vi "Tavle Save for PD.vi"(8 "error in (no error)":errorcluster, 11 "SN":string) -> (0 "error out":errorcluster, 3 "條碼的Index":i32)   [LabVIEW 2019]
uses:
  Ctrl/Table Save.ctl
  LLB/Message/Ctrl/LogType.ctl
  <vilib>/Utility/sysdir.llb/System Directory Type.ctl
  <vilib>/Utility/file.llb/Write Delimited Spreadsheet (string).vi
  LLB/Message/MsgShowAndLog.lvlib
panel:
  out "Read SN Table":string[][](array[string])
  in  "Base Path":path=path "D:/Vicomm"
  out "element":string
  in  "Cluster":cluster{"Table Control":string[][]}={"Table Control"=[["PCBA BARCODE", ""], ["硬體(Tool初始化)", ""], ["company(Tool初始化)", ""], ["耗電流 uA(電流表)", "T"], ["電池負載電壓", "T"], ["晶片ID(Tool FORMAT)", "F"], ["雷雕ID(TOOl scan、藍芽接收器)", "S"], ["Format(Tool FORMAT)", "F"], ["Programe(Tool Programe)", "P"]]}
  # "-1 : 未找到條碼"
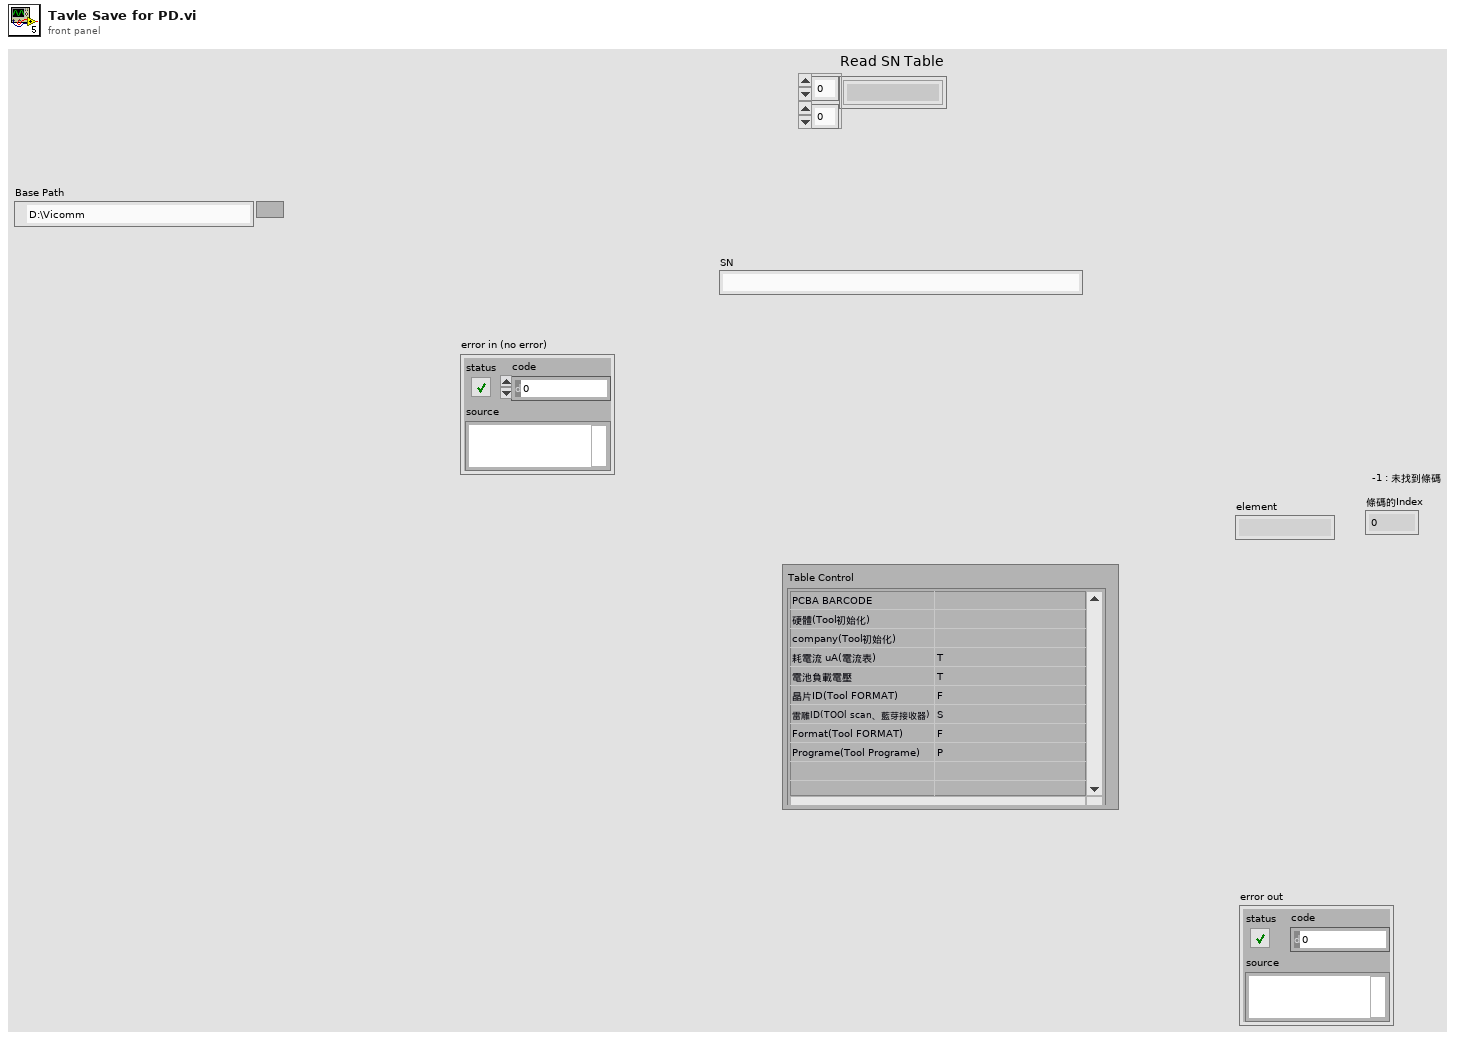
[diagram p1: front panel]
types:
  T1 = typedef "Table Save.ctl" = enum16{"initial", "Add", "Write", "Replace", "Delete", "REad", "RedTable", "Load"}
  T2 = enum16{"open", "replace", "create", "open or create", "replace or create", "replace or create with confirmation"}
  T3 = typedef "MsgShowAndLog.lvlib/LogType.ctl" = enum16{"Auto", "Manual", "Handshake", "Error"}
  T4 = typedef "System Directory Type.ctl" = i32
  T5 = typedef "LVDateTimeRec.ctl" = cluster{"fractional second":dbl, "second":i32, "minute":i32, "hour":i32, "day of month":i32, "month":i32, "year":i32, "day of week":i32, "day of year":i32, "DST":i32}
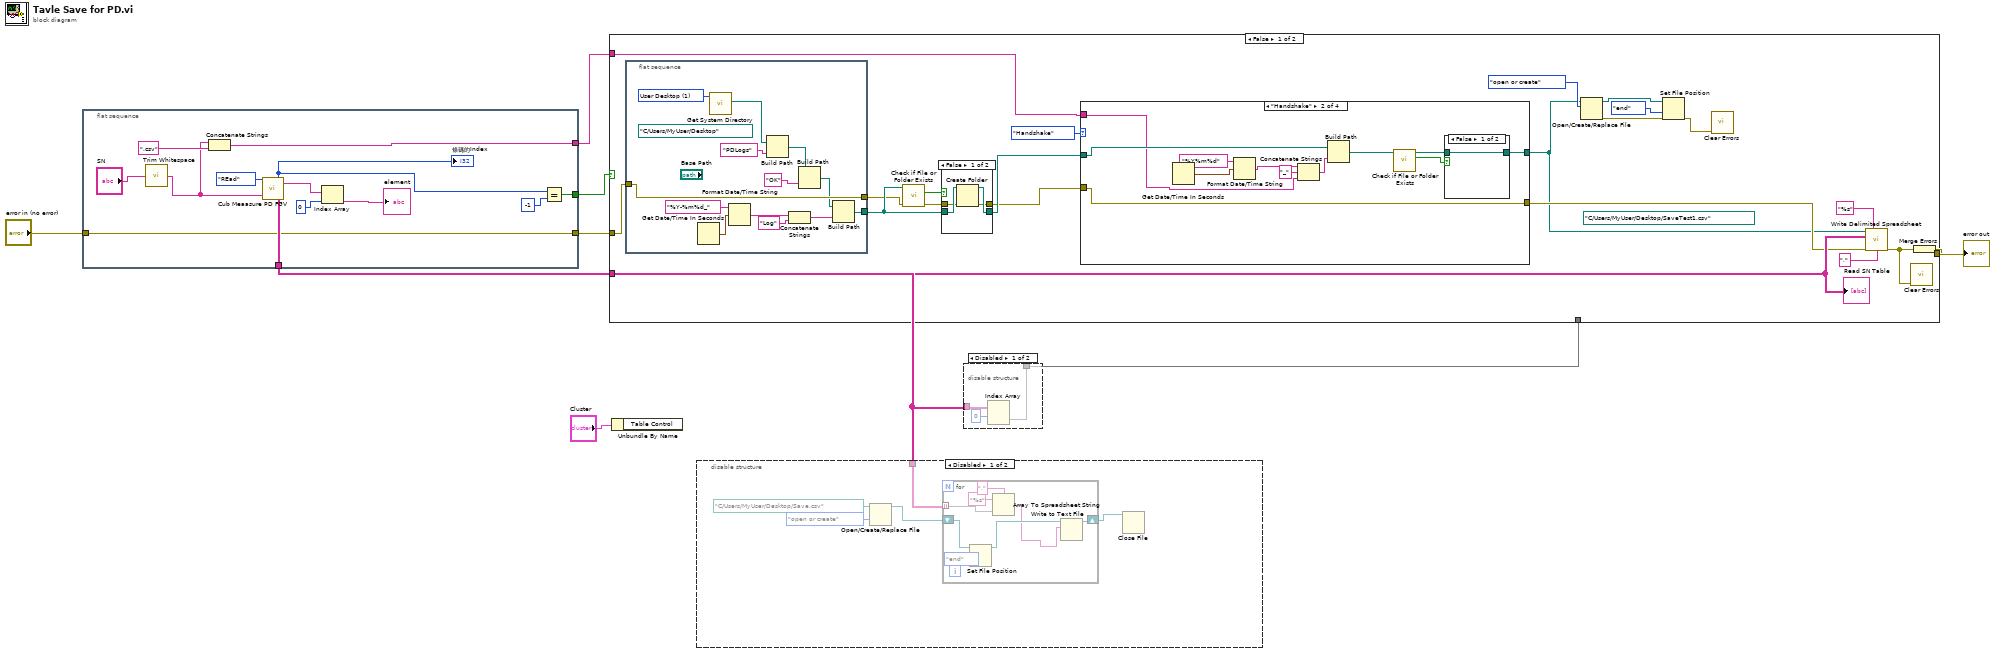
[diagram p0: block diagram]
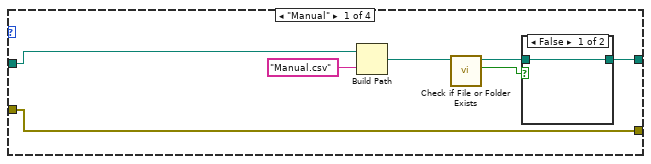
[diagram p2: hidden frame]
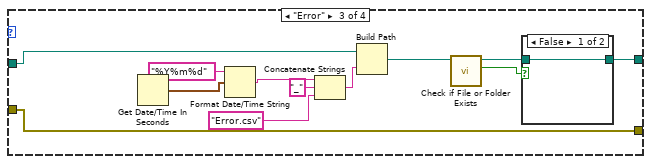
[diagram p5: hidden frame]
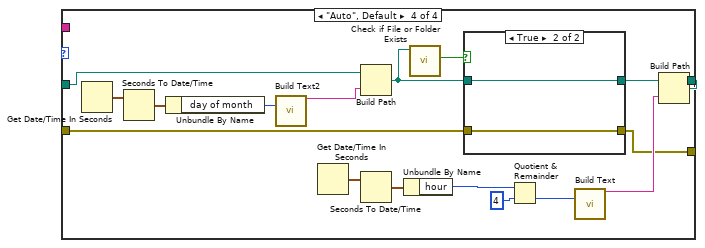
[diagram p7: hidden frame]
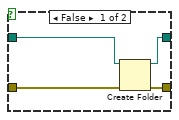
[diagram p8: hidden frame]
diagram:
  n1 = flat-sequence {
    tunnel: [w21] -> w1
    tunnel: [w15] -> w6
    tunnel: "error in (no error)" -> [w12]
    tunnel: [w12] -> w3
    tunnel: [w11] -> w4
    frame #0 {
      n2 = call <vilib>:"Trim Whitespace.vi"("string"="SN") -> ("trimmed string"=w9:string)  [unwired: 1 in]
      n3 = Concatenate Strings(w9, ".csv") -> (w21:string)
      n4 = call "Cub Meaasure PD FGV.vi"("Action"=Table_Save."REad", "SN"=w9) -> ("條碼的Index"=w14:i32, "Read SN Table"=w15:string[][], "Barcode Array"=w17:string[])  [unwired: 10 in, 5 out]
      "條碼的Index" <- w14
      n5 = Index Array(array=w17, index=0) -> (element=→"element":string)
      n6 = Equal?(x=w14, y=-1) -> (x = y?=w11:bool)
    }
  }
  n7 = Unbundle By Name("Cluster") -> ()  [unwired: 1 out]
  n8 = disable-structure shown="Disabled" {
    disable-tunnel: w6 -> [w22 _]
    frame Disabled {
      n9 = Open/Create/Replace File(file path (use dialog)=path "C:/Users/MyUser/Desktop/Save.csv", operation (0:open)=T2."open or create") -> (refnum out=w26:refnum<file>)  [unwired: 4 in, 2 out]
      n10 = for {
        tunnel: w22 -> [w34] mode=indexing
        shift-right: [w31] -> w24
        shift-left: w26 -> [w30]
        n11 = Set File Position(refnum=w30, from (0:start)=enum16{"start", "end", "current"}."end") -> (refnum out=w29:refnum<file>)  [unwired: 2 in, 1 out]
        n12 = Array To Spreadsheet String(delimiter (Tab)=",", array=w34, 3:"%s" ("format string")) -> (spreadsheet string=w27:string)
        n13 = Write to Text File(file (use dialog)=w29, text=w27) -> (refnum out=w31:refnum<file>)  [unwired: 2 in, 2 out]
      }
      n14 = Close File(refnum=w24) -> ()  [unwired: 1 in, 2 out]
    }
    frame Enabled {
    }
  }
  n15 = disable-structure shown="Disabled" {
    disable-tunnel: [w36 _] -> w8
    disable-tunnel: w6 -> [w35 _]
    frame Disabled {
      n16 = Index Array(array=w35, index (row)=0) -> (element=w36:string[])  [unwired: 1 in]
    }
    frame Enabled {
    }
  }
  n17 = case shown="False" w4 {
    tunnel: w8 -> [_ _]
    tunnel: w6 -> [w47 _]
    tunnel: w3 -> [w41 w138]
    tunnel: [w40 w138] -> w2
    tunnel: w1 -> [w39 _]
    frame False {
      (unwired) path "C:/Users/MyUser/Desktop/SaveTest1.csv" ("file path (dialog if empty)")
      n18 = flat-sequence {
        tunnel: [w125] -> w57
        tunnel: w41 -> [w124]
        tunnel: [w124] -> w55
        frame #0 {
          w123 = T4 1 items=["User Home"=0, "User Desktop"=1, "User Documents"=2, "User Application Data"=3, "User Preferences"=4, "User Temporary"=5, "Public Documents"=6, "Public Application Data"=7, "Public Preferences"=8, "Public Cache"=13, "System Core Libraries"=9, "System Installed Libraries"=10, "Application Files"=11, "Boot Volume Root"=12] ("system directory type")
          (unwired) path "C:/Users/MyUser/Desktop" ("file path (dialog if empty)")
          n19 = Get Date/Time In Seconds() -> (seconds since 1Jan1904=w126:timestamp)
          n20 = call <vilib>:"Get System Directory.vi"("system directory type"=w123) -> ("system directory"=w122:path)  [unwired: 10 in]
          n21 = Format Date/Time String(time format string (%c)="%Y-%m%d_", seconds (now)=w126) -> (date/time string=w128:string)  [unwired: 1 in]
          n22 = Build Path(base path=w122, name or relative path="PDLogs") -> (appended path=w120:path)
          n23 = Concatenate Strings(w128, "Log") -> (w130:string)
          n24 = Build Path(base path=w120, name or relative path="OK") -> (appended path=w119:path)
          n25 = Build Path(base path=w119, name or relative path=w130) -> (appended path=w125:path)
        }
      }
      n26 = call <vilib>:"Check if File or Folder Exists.vi"("error in (no error)"=w55, "path"=w57) -> ("error out"=w58:errorcluster, "file or folder exists?"=w56:bool)  [unwired: 7 in, 1 out]
      n27 = case shown="False" w56 {
        tunnel: w57 -> [w135 w137]
        tunnel: [w134 w137] -> w53
        tunnel: w58 -> [w133 w136]
        tunnel: [w132 w136] -> w52
        frame False {
          n28 = Create Folder(path (use dialog)=w135, error in=w133) -> (created path=w134:path, error out=w132:errorcluster)  [unwired: 1 in, 1 out]
        }
        frame True {
        }
      }
      n29 = case shown="\"Handshake\"" LogType."Handshake" ("LogType") {
        tunnel: w53 -> [w65 w79 w93 w107]
        tunnel: w52 -> [w59 w74 w88 w100]
        tunnel: [w60 w75 w89 w99] -> w38
        tunnel: [w59 w74 w88 w96] -> w42
        tunnel: w39 -> [_ w68 _ _]
        frame "Manual" {
          n30 = Build Path(base path=w65, name or relative path="Manual.csv") -> (appended path=w63:path)
          n31 = call <vilib>:"Check if File or Folder Exists.vi"("path"=w63) -> ("file or folder exists?"=w62:bool, "dup path"=w61:path)  [unwired: 8 in, 1 out]
          n32 = case shown="False" w62 {
            tunnel: w61 -> [w66 w67]
            tunnel: [w66 w67] -> w60
            frame False {
            }
            frame True {
            }
          }
        }
        frame "Handshake" {
          n33 = Get Date/Time In Seconds() -> (seconds since 1Jan1904=w73:timestamp)
          n34 = Format Date/Time String(time format string (%c)="%Y%m%d", seconds (now)=w73) -> (date/time string=w70:string)  [unwired: 1 in]
          n35 = Concatenate Strings(w70, "_" ("string"), w68) -> (w71:string)
          n36 = Build Path(base path=w79, name or relative path=w71) -> (appended path=w78:path)
          n37 = call <vilib>:"Check if File or Folder Exists.vi"("path"=w78) -> ("file or folder exists?"=w77:bool, "dup path"=w76:path)  [unwired: 8 in, 1 out]
          n38 = case shown="False" w77 {
            tunnel: w76 -> [w80 w81]
            tunnel: [w80 w81] -> w75
            frame False {
            }
            frame True {
            }
          }
        }
        frame "Error" {
          n39 = Get Date/Time In Seconds() -> (seconds since 1Jan1904=w87:timestamp)
          n40 = Format Date/Time String(time format string (%c)="%Y%m%d", seconds (now)=w87) -> (date/time string=w83:string)  [unwired: 1 in]
          n41 = Concatenate Strings(w83, "_" ("string"), "Error.csv" ("name or relative path")) -> (w85:string)
          n42 = Build Path(base path=w93, name or relative path=w85) -> (appended path=w92:path)
          n43 = call <vilib>:"Check if File or Folder Exists.vi"("path"=w92) -> ("file or folder exists?"=w91:bool, "dup path"=w90:path)  [unwired: 8 in, 1 out]
          n44 = case shown="False" w91 {
            tunnel: w90 -> [w94 w95]
            tunnel: [w94 w95] -> w89
            frame False {
            }
            frame True {
            }
          }
        }
        frame "Auto", Default {
          n45 = Get Date/Time In Seconds() -> (seconds since 1Jan1904=w105:timestamp)
          n46 = Seconds To Date/Time(time stamp (now)=w105) -> (date time rec=w104:T5)  [unwired: 1 in]
          n47 = Unbundle By Name(w104) -> ("day of month"=w106:i32)
          n48 = call "Build Text2"("Date"=w106) -> ("Result"=w103:string)  [unwired: 13 in, 1 out]
          n49 = Get Date/Time In Seconds() -> (seconds since 1Jan1904=w112:timestamp)
          n50 = Build Path(base path=w107, name or relative path=w103) -> (appended path=w98:path)
          n51 = Seconds To Date/Time(time stamp (now)=w112) -> (date time rec=w111:T5)  [unwired: 1 in]
          n52 = Unbundle By Name(w111) -> ("hour"=w109:i32)
          n53 = call <vilib>:"Check if File or Folder Exists.vi"("path"=w98) -> ("file or folder exists?"=w97:bool)  [unwired: 8 in, 2 out]
          n54 = case shown="True" w97 {
            tunnel: w98 -> [w116 w118]
            tunnel: [w115 w118] -> w102
            tunnel: w100 -> [w114 w117]
            tunnel: [w113 w117] -> w96
            frame False {
              n55 = Create Folder(path (use dialog)=w116, error in=w114) -> (created path=w115:path, error out=w113:errorcluster)  [unwired: 1 in, 1 out]
            }
            frame True {
            }
          }
          n56 = Quotient & Remainder(x=w109, y=4) -> (floor(x/y)=w108:i32)  [unwired: 1 out]
          n57 = call "Build Text"("Time"=w108) -> ("Result"=w101:string)  [unwired: 13 in, 1 out]
          n58 = Build Path(base path=w102, name or relative path=w101) -> (appended path=w99:path)
        }
      }
      n59 = Open/Create/Replace File(file path (use dialog)=w38, operation (0:open)=T2."open or create") -> (refnum out=w49:refnum<file>, error out=w51:errorcluster)  [unwired: 4 in, 1 out]
      n60 = Set File Position(refnum=w49, from (0:start)=enum16{"start", "end", "current"}."end", error in=w51) -> (error out=w46:errorcluster)  [unwired: 1 in, 1 out]
      n61 = call <vilib>:"Clear Errors.vi"("error in (no error)"=w46) -> ()  [unwired: 5 in, 2 out]
      n62 = call-poly <vilib>:"Write Delimited Spreadsheet.vi"("file path (dialog if empty)"=w38, "format (%s)"="%s", "2D data"=w47, "error in (no error)"=w42, "delimiter (\\t)"="," ("delimiter (\\t)")) -> ("error out"=w43:errorcluster)  [unwired: 9 in, 1 out]
      n63 = call <vilib>:"Clear Errors.vi"("error in (no error)"=w43) -> ()  [unwired: 5 in, 2 out]
      n64 = Merge Errors(w43) -> (w40:errorcluster)
      "Read SN Table" <- w47
    }
    frame True {
    }
  }
  "error out" <- w2
